vi "Dialogue_UserCredentials.vi"(8 "error in":errorcluster, 11 "Title":string) -> (0 "error out":errorcluster, 1 "Cancelled?":bool, 2 "Password OUT":string, 3 "Username OUT":string)   [LabVIEW 2020, in "hse-ui.lvlib"]
doc: "Shows a dialog window for entering user credentials (username and password).\n\n____\nHAMPEL SOFTWARE ENGINEERING v3.8.0 (2023-12-18 14:41)"
uses:
  hse-ui.lvlib
  FPControl/FPControl_Actions.ctl
panel:
  in  "Password":string
  in  "Username":string
  in  "Btn_Cancel":bool
  in  "Btn_OK":bool
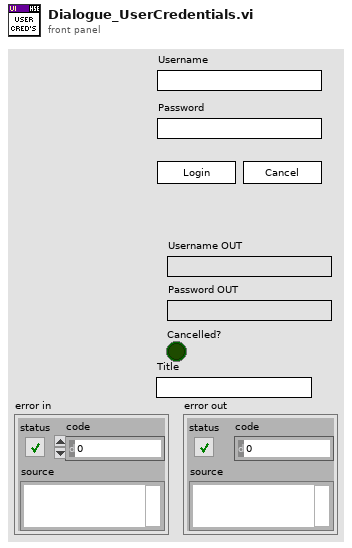
[diagram p1: front panel]
types:
  T1 = typedef "hse-ui.lvlib/FPControl_Actions.ctl" = enum16{"Open", "Hide", "Close", "Bring To Front", "Center", "Minimize", "Maximize"}
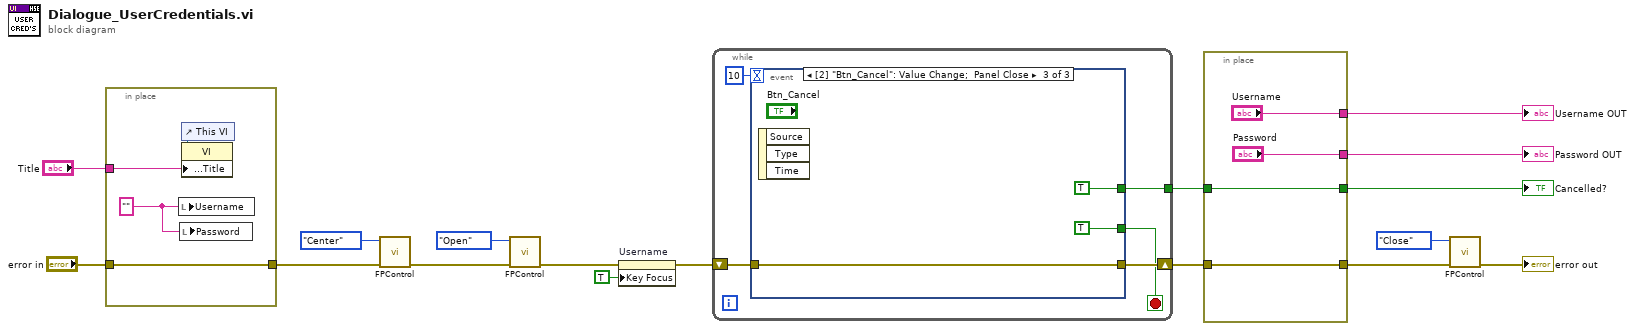
[diagram p0: block diagram]
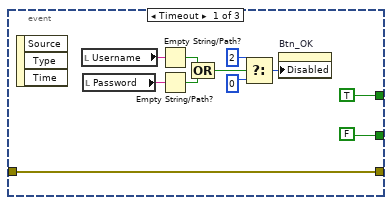
[diagram p2: hidden frame]
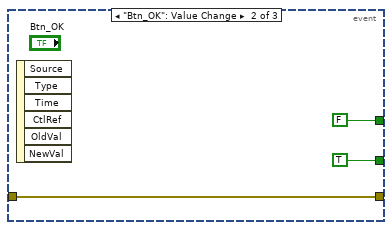
[diagram p3: hidden frame]
diagram:
  n1 = in-place {
    in-place-border: "error in" -> [w20]
    in-place-border: [w20] -> w11
    in-place-border: "Title" -> [w18]
    w21 = "" ("Username")
    n2 = local write "Username"(w21) -> ()
    n3 = local write "Password"(w21) -> ()
    n4 = control-ref of="This VI"() -> (w19:refnum<vi>)
    n5 = property class="VI"(reference=w19, "Front Panel.Title"=w18) -> ()  [unwired: 1 in, 2 out]
  }
  n6 = call "FPControl.vi"("error in"=w11, "Function"=FPControl_Actions."Center") -> ("error out"=w15:errorcluster)  [unwired: 9 out]
  n7 = call "FPControl.vi"("error in"=w15, "Function"=FPControl_Actions."Open") -> ("error out"=w9:errorcluster)  [unwired: 9 out]
  n8 = property on="Username" class="Str"(error in=w9, "Key Focus"=TRUE) -> (error out=w8:errorcluster)  [unwired: 1 in, 1 out]
  n9 = while {
    shift-right: [w24] -> w7
    shift-left: w8 -> [w25]
    tunnel: [w22] -> w4
    stop <- w23 stop-if-true
    n10 = event shown="[2] \"Btn_Cancel\": Value Change;  Panel Close" {
      selector: _ -> [_ _ _]
      dyn-events: _ -> [_ _ _]
      timeout: 10 -> [_ _ _]
      tunnel: w25 -> [w36 w40 w43]
      tunnel: [w36 w40 w43] -> w24
      tunnel: [FALSE TRUE TRUE] -> w23
      tunnel: [TRUE FALSE TRUE] -> w22
      event Timeout {
        n11 = event-data() -> ()  [unwired: 1 in, 3 out]
        n12 = local read "Username"() -> (w31:string)
        n13 = local read "Password"() -> (w32:string)
        n14 = Empty String/Path?(string/path=w31) -> (empty?=w30:bool)
        n15 = Empty String/Path?(string/path=w32) -> (empty?=w29:bool)
        n16 = Compound Arithmetic op=OR(w30, w29) -> (w28:bool)
        n17 = Select(t=u8 2 ("Disabled"), s=w28, f=u8 0 ("Disabled")) -> (s? t:f=w35:u8)
        n18 = property on="Btn_OK" class="Bool"("Disabled"=w35) -> ()  [unwired: 2 in, 2 out]
      }
      event "Btn_OK": Value Change {
        n19 = event-data() -> ()  [unwired: 1 in, 6 out]
      }
      event "Btn_Cancel": Value Change; Panel Close {
        n20 = event-data() -> ()  [unwired: 1 in, 3 out]
      }
    }
  }
  n21 = in-place {
    in-place-border: w7 -> [w47]
    in-place-border: [w47] -> w6
    in-place-border: [w46] -> w5
    in-place-border: w4 -> [w46]
    in-place-border: ["Username"] -> w3
    in-place-border: ["Password"] -> w2
  }
  "Cancelled?" <- w5
  "Username OUT" <- w3
  "Password OUT" <- w2
  n22 = call "FPControl.vi"("error in"=w6, "Function"=FPControl_Actions."Close") -> ("error out"=→"error out":errorcluster)  [unwired: 9 out]
